vi "_createKafkaEvents - Copy.vi"(0 "Payload":string[](array[string]), 3 "error in (no error)":errorcluster) -> (7 "Kafka Events":T1[](array[typedef]), 10 "error out":errorcluster)   [LabVIEW 2019]
uses:
  KafkaLVLib/API/KafkaConsumerEvent.ctl
  1f099e04-d0a3-4231-929c-9bf0d6f2adbc.vi
  <vilib>/JDP Science/JSONtext/String Subset.vi
  <vilib>/JDP Science/JSONtext/Parsing/Parse Full Path or Item Name.vi
  <vilib>/JDP Science/JSONtext/Next JSON Value.vi
  <vilib>/JDP Science/JSONtext/support/Error Cluster From Code.vi
  <vilib>/JDP Science/JSONtext/Offset/Find Item Locations by Path.vi
  <vilib>/JDP Science/JSONtext/JSON text to Variant.vi
  <vilib>/JDP Science/JSONtext/JSONtext.lvlib
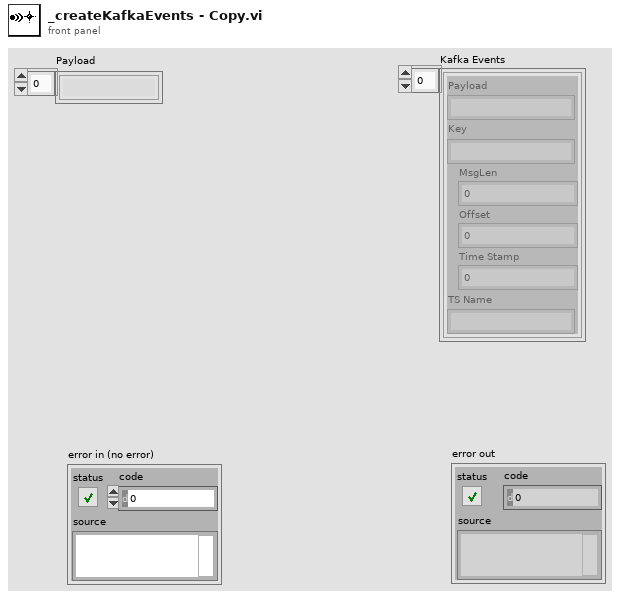
[diagram p1: front panel]
types:
  T1 = typedef "KafkaConsumerEvent.ctl" = cluster{"Payload":string, "Key":string, "MsgLen":u64, "Offset":i64, "Time Stamp":i64, "TS Name":string}
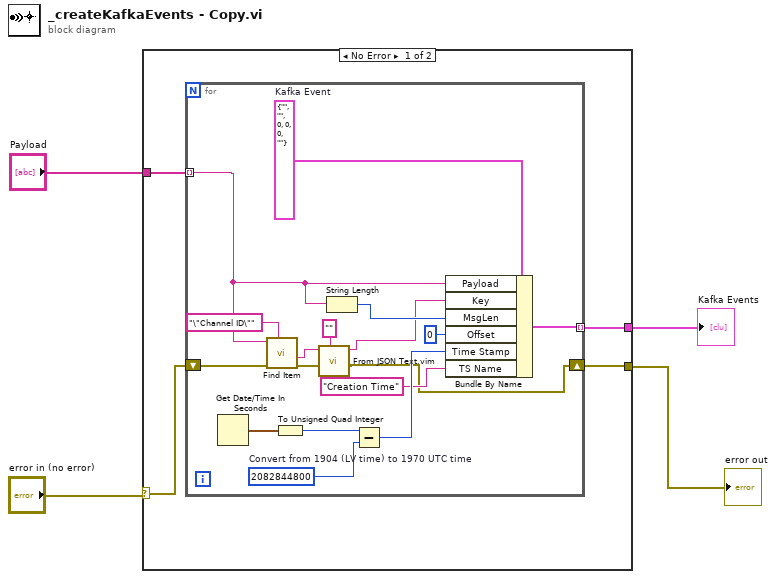
[diagram p0: block diagram]
diagram:
  n1 = case shown="No Error" "error in (no error)" {
    selector: "error in (no error)" -> [w7 w26]
    tunnel: "Payload" -> [w8 _]
    tunnel: [w6 w26] -> w2
    tunnel: [w5 _] -> w1
    frame No Error {
      n2 = for {
        tunnel: w8 -> [w22] mode=indexing
        shift-right: [w9] -> w6
        shift-left: w7 -> [w23]
        tunnel: [w14] -> w5 mode=indexing
        w18 = u64 2082844800  # Convert from 1904 (LV time) to 1970 UTC time
        w25 = T1 {"Payload"="", "Key"="", "MsgLen"=0, "Offset"=0, "Time Stamp"=0, "TS Name"=""}  # Kafka Event
        n3 = Get Date/Time In Seconds() -> (seconds since 1Jan1904=w20:timestamp)
        n4 = call <vilib>:"Find Item.vi"("$Path or Item Name"="\"Channel ID\"", "error in (no error)"=w23, "JSON"=w22) -> ("error out"=w17:errorcluster, "<JSON>"=w12:string)  [unwired: 5 in, 2 out]
        n5 = To Unsigned Quad Integer(1:w20) -> (0:w19:u64)
        n6 = call "From JSON Text.vim"("Data Type and Default Value"="", "error in (no error)"=w17, "JSON"=w12) -> ("error out"=w9:errorcluster, "Data out"=w10:string)  [unwired: 7 in]
        n7 = String Length(string=w22) -> (length=w21:i32)
        n8 = Subtract(x=w19, y=w18) -> (x-y=w16:u64)
        n9 = Bundle By Name(cluster=w25, "Payload"=w22, "Key"=w10, "MsgLen"=w21, "Offset"=i64 0, "Time Stamp"=w16, "TS Name"="Creation Time") -> (w14:T1)
      }
    }
    frame Error {
    }
  }
  "error out" <- w2
  "Kafka Events" <- w1
